vi "DecodeFromFile.vi"() -> ()   [LabVIEW 2020]
panel:
  out "Image":T1(plugin-control)
  out "error":errorcluster
  in  "Pixel Format":enum16{"RAW12_GR", "YUV422"}(ring)
  in  "Height":i32=2168
  in  "Width":i32=3848
  in  "file (use dialog)":path
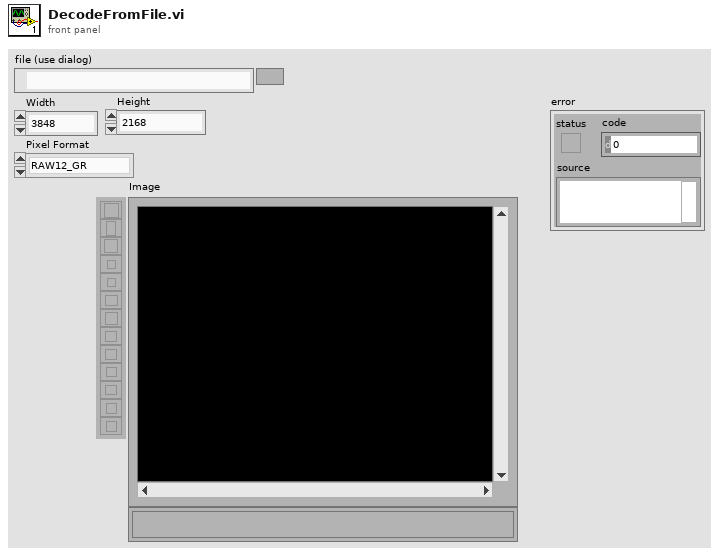
[diagram p1: front panel]
types:
  T1 = typedef "IMAQ Image.ctl" = refnum<image>
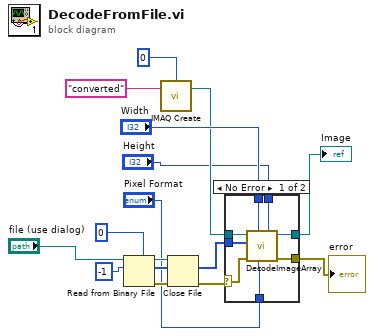
[diagram p0: block diagram]
diagram:
  n1 = Read from Binary File(5:u8 0, 10:-1 ("count (1)"), 11:"file (use dialog)") -> (0:w5:errorcluster, 2:w6:u8[], 3:w4:refnum<file>)  [unwired: 3 in, 1 out]
  n2 = call "IMAQ Create"("Border Size"=0, "Image Name"="converted") -> ("New Image"=w7:T1)  [unwired: 3 in, 1 out]
  n3 = Close File(refnum=w4, error in=w5) -> (error out=w3:errorcluster)  [unwired: 1 out]
  n4 = case shown="No Error" w3 {
    selector: w3 -> [w18 w25]
    tunnel: "Width" -> [w23 _]
    tunnel: [w22 w24] -> w11
    tunnel: [w21 w25] -> w10
    tunnel: w7 -> [w20 w24]
    tunnel: w6 -> [w19 _]
    tunnel: "Height" -> [w17 _]
    tunnel: "Pixel Format" -> [w16 _]
    frame No Error {
      n5 = call "DecodeImageArray.vi"("Height"=w17, "Pixel Format"=w16, "Width"=w23, "error in (no error)"=w18, "Array"=w19, "image  in"=w20) -> ("error out"=w21:errorcluster, "image out"=w22:T1)  [unwired: 4 in]
    }
    frame Error {
    }
  }
  "Image" <- w11
  "error" <- w10
